vi "Configuration 1.1 JSON Unflatten.vi"(8 "error in (no error)":errorcluster, 11 "dsf configuration json":string) -> (0 "error out":errorcluster, 3 "framework configuration 1.1":T1={"plugins"=[{"name"="Plugin", "components"=[], "cycle timing"={"priority"=10000, "decimation"=1, "offset"=0}, "threads"=[], "transfer groups"=[{"name"="Group", "direction"=0, "cycle timing"={"priority"=100, "decimation"=1, "offset"=0}, "thread index"=-1, "settings"=[], "transfers"=[{"name"="Transfer", "byte order"=0, "settings"=[], "channels"=[{"string offset"=0, "string data type"=2, "engine data type"=2, "name"="Channel", "settings"=[], "units"="V"}]}], "timeout behavior"=0}], "settings"=[]}]})   [LabVIEW 2021, in "DSF Core.lvlib" / "Configuration Session.lvclass"]
uses:
  Configuration Session.lvclass
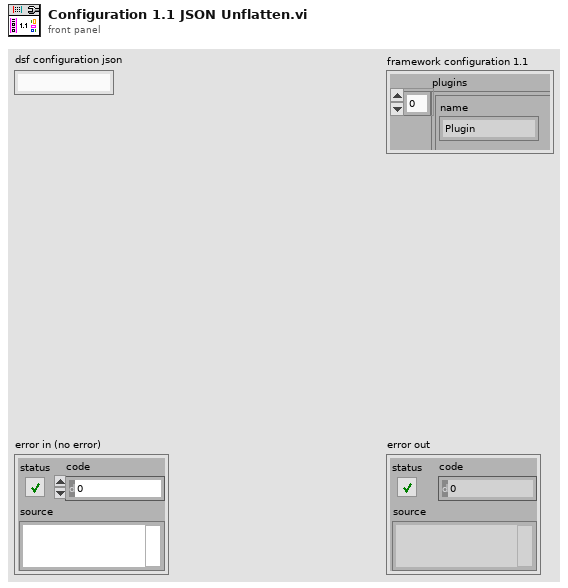
[diagram p1: front panel]
types:
  T1 = cluster{"plugins":cluster{"name":string, "components":string[], "cycle timing":cluster{"priority":u64, "decimation":u64, "offset":u64}, "threads":cluster{"buffer converter settings":cluster{"key":string, "value":string}[], "transceiver settings":cluster{"key":string, "value":string}[], "custom settings":cluster{"key":string, "value":string}[], "processor":i32, "priority offset":i16}[], "transfer groups":cluster{"name":string, "direction":u8, "cycle timing":cluster{"priority":u64, "decimation":u64, "offset":u64}, "thread index":i32, "settings":cluster{"key":string, "value":string}[], "transfers":cluster{"name":string, "byte order":u8, "settings":cluster{"key":string, "value":string}[], "channels":cluster{"string offset":u64, "string data type":u8, "engine data type":u8, "name":string, "settings":cluster{"key":string, "value":string}[], "units":string}[]}[], "timeout behavior":u8}[], "settings":cluster{"key":string, "value":string}[]}[]}
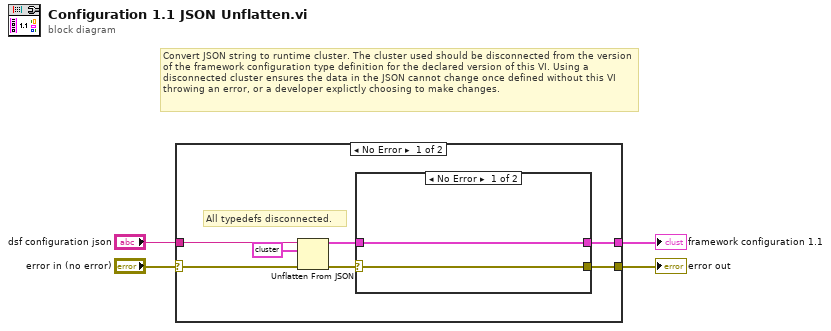
[diagram p0: block diagram]
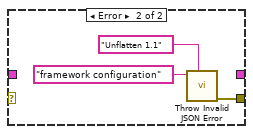
[diagram p2: hidden frame]
diagram:
  # "Convert JSON string to runtime cluster. The cluster used should be disconnected from the version of the framework configuration type definition for the declared version of this VI. Using a disconnected cluster ensures the data in the JSON cannot change once defined without this VI throwing an error, or a developer explictly choosing to make changes."
  n1 = case shown="No Error" "error in (no error)" {
    selector: "error in (no error)" -> [w7 w17]
    tunnel: "dsf configuration json" -> [w6 _]
    tunnel: [w10 w17] -> w3
    tunnel: [w8 _] -> w1
    frame No Error {
      # "All typedefs disconnected."
      n2 = Unflatten From JSON(JSON string=w6, type and defaults=T1 {"plugins"=[{"name"="Plugin", "components"=["UDP"], "cycle timing"={"priority"=10000, "decimation"=1, "offset"=0}, "threads"=[{"buffer converter settings"=[{"key"="a", "value"="a"}], "transceiver settings"=[{"key"="a", "value"="a"}], "custom settings"=[{"key"="a", "value"="a"}], "processor"=-2, "priority offset"=0}], "transfer groups"=[{"name"="Group", "direction"=0, "cycle timing"={"priority"=100, "decimation"=1, "offset"=0}, "thread index"=-1, "settings"=[{"key"="a", "value"="a"}], "transfers"=[{"name"="Transfer", "byte order"=0, "settings"=[{"key"="a", "value"="a"}], "channels"=[{"string offset"=0, "string data type"=2, "engine data type"=2, "name"="Channel", "settings"=[{"key"="a", "value"="a"}], "units"="V"}]}], "timeout behavior"=0}], "settings"=[{"key"="a", "value"="a"}]}]} ("framework configuration 1.1"), error in (no error)=w7) -> (value=w9:T1, error out=w11:errorcluster)  [unwired: 4 in]
      n3 = case shown="No Error" w11 {
        selector: w11 -> [w13 _]
        tunnel: [w13 w16] -> w10
        tunnel: w9 -> [w12 _]
        tunnel: [w12 _] -> w8
        frame No Error {
        }
        frame Error {
          n4 = call "Throw Invalid JSON Error.vi"("error source vi name"="Unflatten 1.1", "name"="framework configuration") -> ("error out"=w16:errorcluster)  [unwired: 9 in]
        }
      }
    }
    frame Error {
    }
  }
  "error out" <- w3
  "framework configuration 1.1" <- w1
